vi "Register.vi"(0 "WAMP Client in":refnum<class "WAMP Client.lvclass">, 1 "Options":string, 5 "Procedure URI":string, 7 "INVOCATION event":refnum<user-event>, 11 "error in (no error)":errorcluster) -> (4 "WAMP Client out":refnum<class "WAMP Client.lvclass">, 6 "Success?":bool, 8 "WAMP Error":T1, 15 "error out":errorcluster)   [LabVIEW 2020, in "WAMP Client.lvclass"]
uses:
  <userlib>/lvwamp/WAMP Client/WAMP Client.lvclass
  <userlib>/lvwamp/WAMP Client/WAMP Client.lvclass/WAMP Client.ctl
  <userlib>/lvwamp/WAMP Client/TypeDef/WAMP Error Payload.ctl
  <userlib>/lvwamp/WAMP Client/TypeDef/REGISTERED or ERROR payload.ctl
  <vilib>/ErrorRing/Error Ring.xnode
  <vilib>/Utility/error.llb/Error Cluster From Error Code.vi
  <userlib>/lvwamp/WAMP Client/TypeDef/INVOCATION payload.ctl
panel:
  in  "Time Out (ms) (-1)":i32
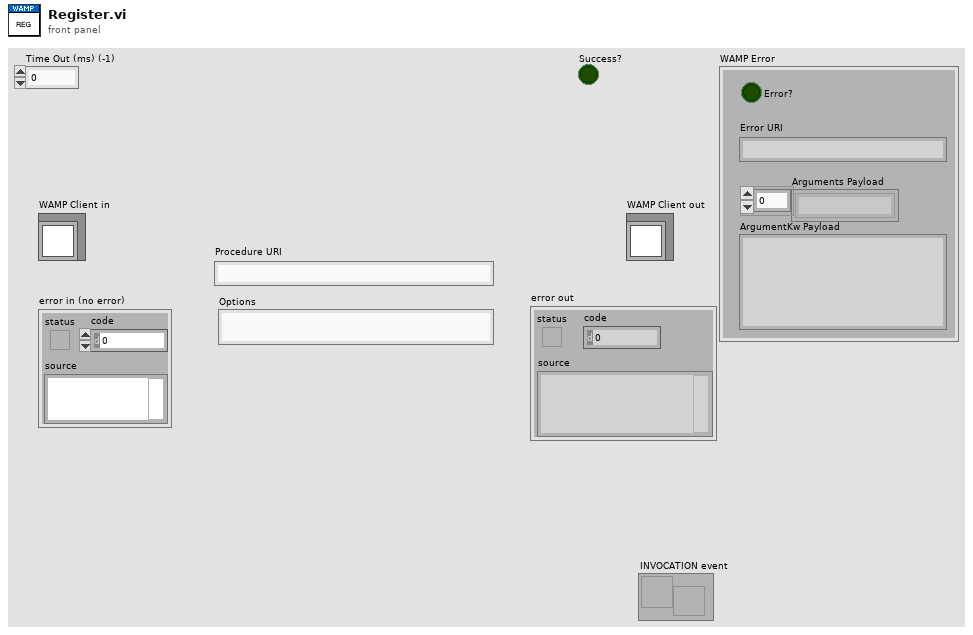
[diagram p1: front panel]
types:
  T1 = typedef "WAMP Client.lvclass/WAMP Error Payload.ctl" = cluster{"Arguments Payload":string[], "ArgumentKw Payload":string, "Error URI":string, "Error?":bool}
  T2 = typedef "WAMP Client.lvclass/REGISTERED or ERROR payload.ctl" = cluster{"Register Request ID":u32, "Registration ID":u32, "Success?":bool, "WAMP Error":T1, "Procedure URI":string}
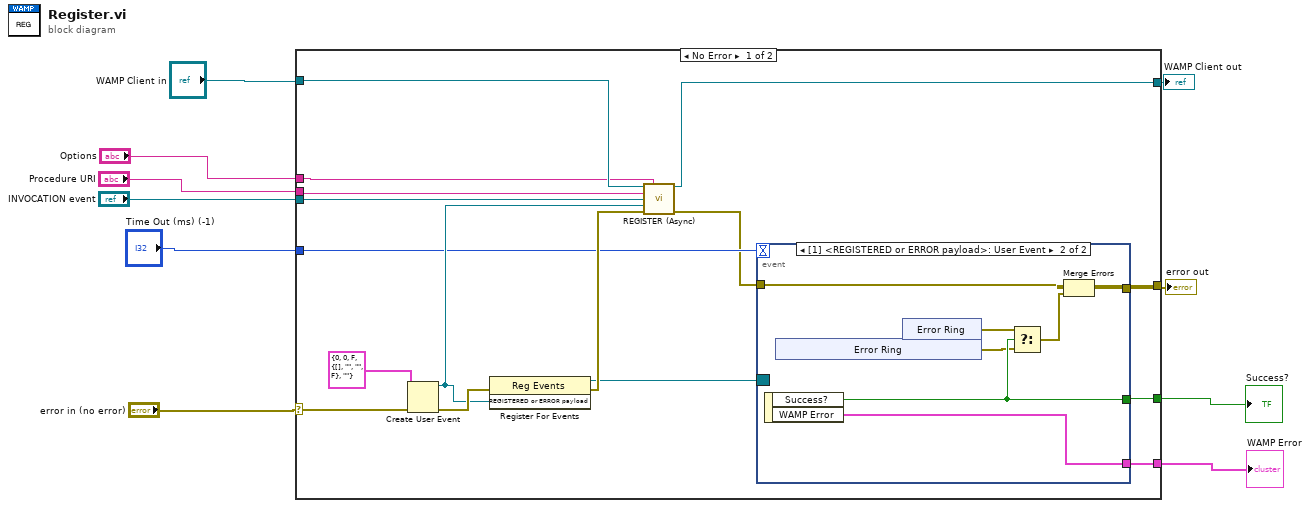
[diagram p0: block diagram]
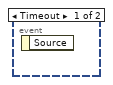
[diagram p2: hidden frame]
diagram:
  n1 = case shown="No Error" "error in (no error)" {
    selector: "error in (no error)" -> [w21 w41]
    tunnel: [w11 w41] -> w9
    tunnel: [w15 w40] -> w7
    tunnel: "WAMP Client in" -> [w26 w40]
    tunnel: "Procedure URI" -> [w25 _]
    tunnel: "Options" -> [w24 _]
    tunnel: "INVOCATION event" -> [w23 _]
    tunnel: "Time Out (ms) (-1)" -> [w16 _]
    tunnel: [w14 _] -> w2
    tunnel: [w13 _] -> w1
    frame No Error {
      n2 = Create User Event(user event datatype=T2 {"Register Request ID"=0, "Registration ID"=0, "Success?"=FALSE, "WAMP Error"={"Arguments Payload"=[], "ArgumentKw Payload"="", "Error URI"="", "Error?"=FALSE}, "Procedure URI"=""} ("REGISTERED or ERROR payload"), error in=w21) -> (user event=w19:refnum<user-event>, error out=w20:errorcluster)
      n3 = register-events(error in=w20, w19) -> (reference out=w17:refnum<event-registration>, error out=w18:errorcluster)  [unwired: 1 in]
      n4 = call-dynamic "REGISTER (Async).vi"("WAMP Client in"=w26, "Options"=w24, "Procedure URI"=w25, "INVOCATION event"=w23, "REGISTERED or ERROR event"=w19, "error in (no error)"=w18) -> ("WAMP Client out"=w15:refnum<class "WAMP Client.lvclass">, "error out"=w12:errorcluster)  [unwired: 8 in]
      n5 = event shown="[1] <REGISTERED or ERROR payload>: User Event" {
        selector: w17 -> [_ _]
        dyn-events: _ -> [_ _]
        timeout: w16 -> [_ _]
        tunnel: [_ w30] -> w14
        tunnel: [_ w33] -> w13
        tunnel: w12 -> [_ w32]
        tunnel: [_ w31] -> w11
        event Timeout {
          n6 = event-data() -> ()  [unwired: 1 in, 1 out]
        }
        event User Event {
          n7 = event-data() -> ("Success?"=w30:bool, "WAMP Error"=w33:T1)  [unwired: 1 in]
          n8 = xnode "Error Ring"() -> ("error out"=w28:errorcluster)
          n9 = xnode "Error Ring"() -> ("error out"=w29:errorcluster)
          n10 = Select(t=w29, s=w30, f=w28) -> (s? t:f=w27:errorcluster)
          n11 = Merge Errors(w32, w27) -> (w31:errorcluster)
        }
      }
    }
    frame Error {
    }
  }
  "error out" <- w9
  "WAMP Client out" <- w7
  "Success?" <- w2
  "WAMP Error" <- w1
